vi "Correlation_M2.vi"() -> ()   [LabVIEW 2015]
uses:
  <vilib>/Analysis/NI_AALBase.lvlib
panel:
  out "shift register out D":dbl[](array[numeric])
  in  "shift register D":dbl[](array[numeric])=[0.0, 0.0, 0.0, 0.0, 0.0, 0.0, 0.0, 0.0, 0.0, 0.0, 0.0, 0.0, 0.0, 0.0, 0.0, 0.0, 0.0, 0.0, 0.0, 0.0, 0.0, 0.0, 0.0, 0.0, 0.0, 0.0, 0.0, 0.0, 0.0, 0.0, 0.0, 0.0, 0.0, 0.0, 0.0, 0.0, 0.0, 0.0, 0.0, 0.0, 0.0, 0.0, 0.0, 0.0, 0.0, 0.0, 0.0, 0.0, 0.0, 0.0, 0.0, 0.0, 0.0, 0.0, 0.0, 0.0, 0.0, 0.0, 0.0, 0.0, 0.0, 0.0, 0.0, 0.0]
  out "MnB":dbl[](array[numeric])
  in  "Input B":dbl[](array[numeric])=[1.0, 2.0, 5.0, 0.0, 10.0, 1.0, 4.0, 1.0, 2.0]
  out "shift register Y out":dbl[](array[numeric])
  in  "shift register MY":dbl[](array[numeric])=[0.0, 0.0, 0.0, 0.0, 0.0, 0.0, 0.0, 0.0, 0.0]
  in  "m":i32=3
  out "MnA":dbl[](array[numeric])
  in  "Acc in":dbl[](array[numeric])=[0.0, 0.0, 0.0, 0.0, 0.0, 0.0, 0.0, 0.0, 0.0]
  in  "shift register in":dbl[](array[numeric])=[0.0, 0.0, 0.0, 0.0, 0.0, 0.0, 0.0, 0.0, 0.0]
  in  "Input A":dbl[](array[numeric])=[1.0, 2.0, 5.0, 0.0, 10.0, 1.0, 4.0, 1.0, 2.0]
  out "Acc":dbl[](array[numeric]) format="%#_10g"
  out "shift register":dbl[](array[numeric])
  out "New Mn":bool=TRUE
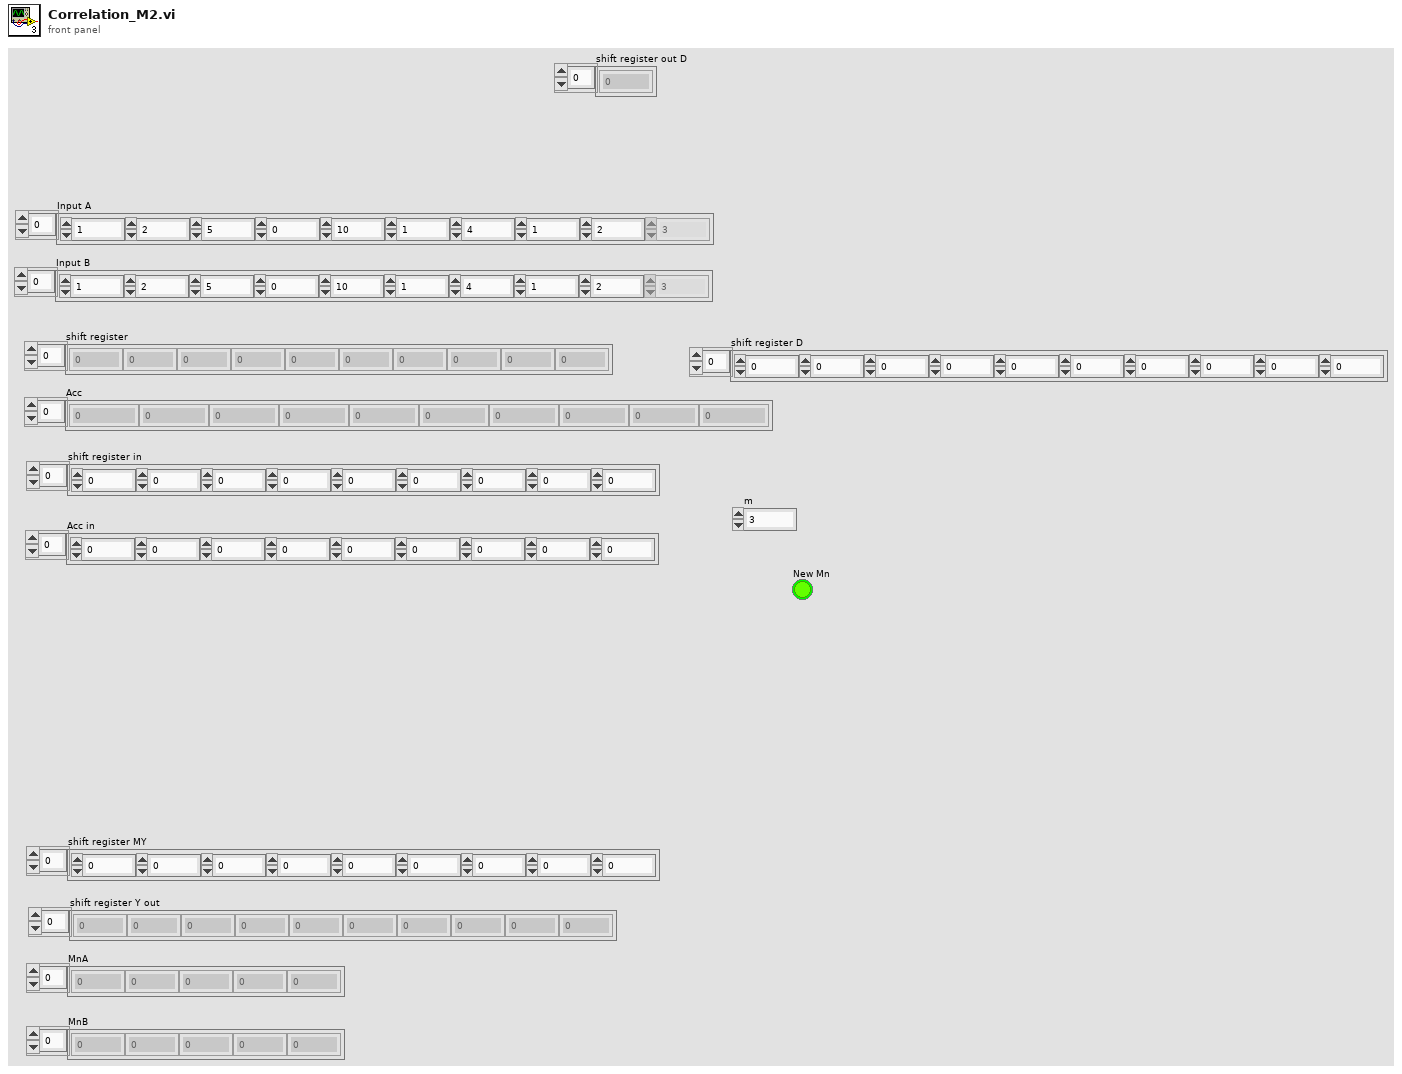
[diagram p1: front panel]
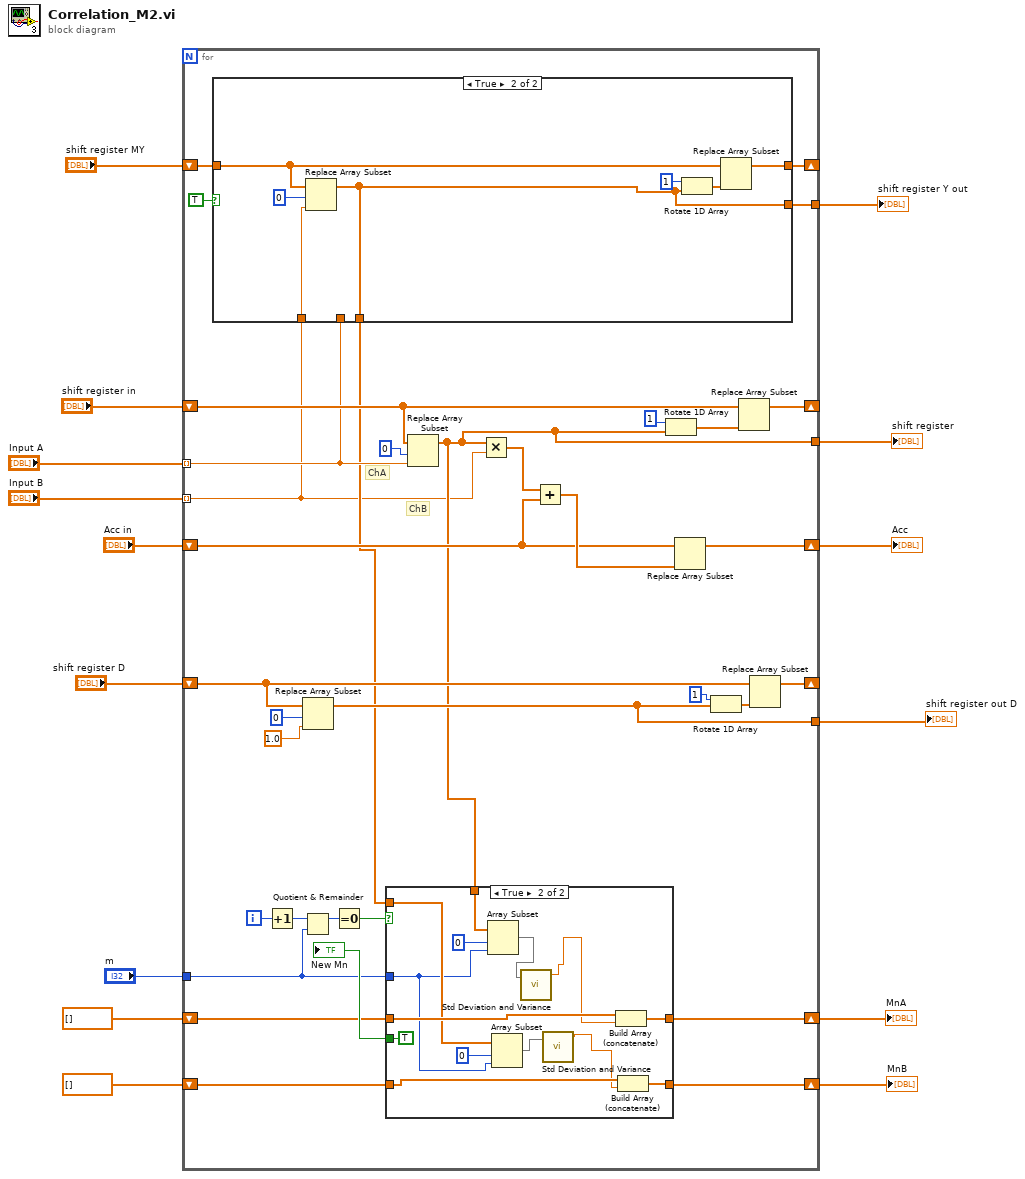
[diagram p0: block diagram]
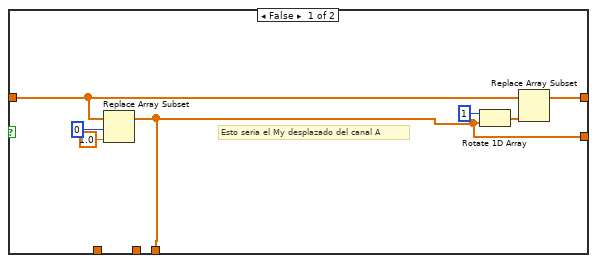
[diagram p2: hidden frame]
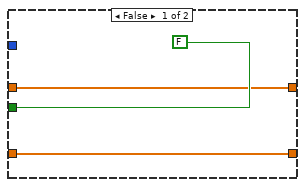
[diagram p3: hidden frame]
diagram:
  n1 = for {
    tunnel: "Input A" -> [w29] mode=indexing
    shift-right: [w45] -> _
    shift-left: "shift register in" -> [w34]
    shift-right: [w43] -> w1
    shift-left: "Acc in" -> [w44]
    tunnel: [w18] -> w15
    shift-right: [w37] -> w4
    shift-left: dbl[] [] -> [w38]
    tunnel: "m" -> [w36]
    shift-right: [w33] -> _
    shift-left: "shift register MY" -> [w32]
    tunnel: [w31] -> w8
    tunnel: "Input B" -> [w16] mode=indexing
    shift-right: [w27] -> w5
    shift-left: dbl[] [] -> [w28]
    shift-right: [w20] -> _
    shift-left: "shift register D" -> [w21]
    tunnel: [w19] -> w2
    i -> [w30]
    # "ChA"
    # "ChB"
    n2 = case shown="True" TRUE {
      tunnel: [w52 w59] -> w33
      tunnel: w32 -> [w51 w60]
      tunnel: [w50 w57] -> w31
      tunnel: w29 -> [_ _]
      tunnel: w16 -> [_ w58]
      tunnel: [w50 w57] -> w17
      frame False {
        # "Esto seria el My desplazado del canal A"
        n3 = Replace Array Subset(array=w51, new element=sgl 1.0 ("new element/subarray"), index=0) -> (w50:dbl[])
        n4 = Rotate 1D Array(1:w50, 2:1 ("n")) -> (0:w53:dbl[])
        n5 = Replace Array Subset(array=w51, new element=w53) -> (w52:dbl[])  [unwired: 1 in]
      }
      frame True {
        n6 = Replace Array Subset(array=w60, new element=w58, index=0) -> (w57:dbl[])
        n7 = Rotate 1D Array(1:w57, 2:1 ("n")) -> (0:w61:dbl[])
        n8 = Replace Array Subset(array=w60, new element=w61) -> (w59:dbl[])  [unwired: 1 in]
      }
    }
    n9 = Increment(x=w30) -> (x+1=w41:i32)
    n10 = Replace Array Subset(array=w21, new element=sgl 1.0 ("new element/subarray"), index=0) -> (w19:dbl[])
    n11 = Quotient & Remainder(x=w41, y=w36) -> (x-y*floor(x/y)=w40:i32)  [unwired: 1 out]
    n12 = Equal To 0?(x=w40) -> (x = 0?=w39:bool)
    n13 = Replace Array Subset(array=w34, new element=w29, index=0) -> (w18:dbl[])
    n14 = case shown="True" w39 {
      tunnel: w18 -> [_ w80]
      tunnel: [FALSE TRUE] -> w42
      tunnel: w36 -> [_ w71]
      tunnel: w38 -> [w65 w78]
      tunnel: [w65 w77] -> w37
      tunnel: w28 -> [w64 w74]
      tunnel: [w64 w75] -> w27
      tunnel: w17 -> [_ w72]
      frame False {
      }
      frame True {
        n15 = Array Subset(array=w80, index=0, length=w71) -> (w70:dbl[])
        n16 = Array Subset(array=w72, index=0, length=w71) -> (w68:dbl[])
        n17 = call <vilib>:"Std Deviation and Variance.vi"("X"=w70) -> ("mean"=w69:dbl)  [unwired: 1 in, 2 out]
        n18 = call <vilib>:"Std Deviation and Variance.vi"("X"=w68) -> ("mean"=w67:dbl)  [unwired: 1 in, 2 out]
        n19 = Build Array (concatenate)(w78, w69) -> (w77:dbl[])
        n20 = Build Array (concatenate)(w74, w67) -> (w75:dbl[])
      }
    }
    "New Mn" <- w42
    n21 = Multiply(x=w18, y=w16) -> (x*y=w48:dbl[])
    n22 = Add(x=w48, y=w44) -> (x+y=w47:dbl[])
    n23 = Rotate 1D Array(1:w18, 2:1 ("n")) -> (0:w35:dbl[])
    n24 = Replace Array Subset(array=w44, new element=w47) -> (w43:dbl[])  [unwired: 1 in]
    n25 = Rotate 1D Array(1:w19, 2:1 ("n")) -> (0:w22:dbl[])
    n26 = Replace Array Subset(array=w34, new element=w35) -> (w45:dbl[])  [unwired: 1 in]
    n27 = Replace Array Subset(array=w21, new element=w22) -> (w20:dbl[])  [unwired: 1 in]
  }
  "shift register" <- w15
  "Acc" <- w1
  "MnA" <- w4
  "shift register Y out" <- w8
  "MnB" <- w5
  "shift register out D" <- w2
